vi "createNetworkConnection.vi"(8 "error in (no error)":errorcluster, 11 "BuildWorker in":refnum<class "BuildWorker.lvclass">) -> (0 "error out":errorcluster, 3 "BuildWorker out":refnum<class "BuildWorker.lvclass">)   [LabVIEW 2017, in "BuildWorker.lvlib" / "BuildWorker.lvclass"]
uses:
  BuildWorker.lvclass
  C:/Program Files (x86)/National Instruments/LabVIEW 2017/vi.lib/ActorFramework/Actor/Actor.lvclass
  BuildWorker Messages/New Message Msg/New Message Msg.lvclass
  C:/Users/Public/Documents/wc/BuildFarm/src/LabVIEW/vi.lib/BenjaminR/Build Farm/Actors/Communication/WebSocket Client/WebSocket Client Messages/New Message Msg/New Message Msg.lvclass
  BuildWorker.lvclass/BuildWorker.ctl
  Communication/WebSocket Client/WebSocket Client/WebSocket Client.lvclass/WebSocket Client.ctl
  Communication/WebSocket Client/WebSocket Client/WebSocket Client.lvclass
  <vilib>/ActorFramework/Actor/Actor.lvclass
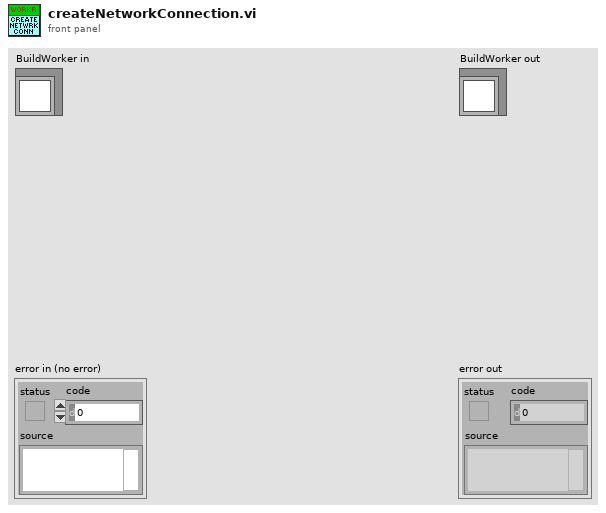
[diagram p1: front panel]
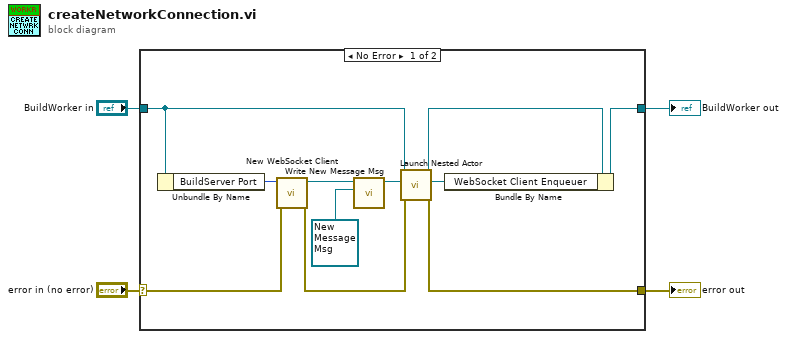
[diagram p0: block diagram]
diagram:
  n1 = case shown="No Error" "error in (no error)" {
    selector: "error in (no error)" -> [w14 w17]
    tunnel: [w8 w17] -> w3
    tunnel: [w15 w16] -> w1
    tunnel: "BuildWorker in" -> [w12 w16]
    frame No Error {
      n2 = Unbundle By Name(w12) -> ("BuildServer Port"=w13:u16)
      n3 = call "New WebSocket Client.vi"("error in (no error)"=w14, "Port"=w13) -> ("error out"=w10:errorcluster, "WebSocket Client out"=w7:refnum<class "WebSocket Client.lvclass">)  [unwired: 8 in]
      n4 = call "Write New Message Msg.vi"("WebSocket Client.lvlib:New Message Msg.lvclass"=refnum<class "New Message Msg.lvclass"> refnum ("BuildWorker.lvlib:New Message Msg.lvclass"), "WebSocket Client in"=w7) -> ("WebSocket Client out"=w6:refnum<class "WebSocket Client.lvclass">)  [unwired: 9 in]
      n5 = call <vilib>:"Launch Nested Actor.vi"("error in (no error)"=w10, "Nested Actor"=w6, "Caller Actor in"=w12) -> ("error out"=w8:errorcluster, "Nested Actor's Enqueuer"=w9:refnum<class "Message Enqueuer.lvclass">, "Caller Actor out"=w11:refnum<class "BuildWorker.lvclass">)  [unwired: 6 in]
      n6 = Bundle By Name(cluster=w11, "WebSocket Client Enqueuer"=w9) -> (w15:refnum<class "BuildWorker.lvclass">)
    }
    frame Error {
    }
  }
  "error out" <- w3
  "BuildWorker out" <- w1
